vi "Lot_Unload.vi"(8 "error in (no error)":errorcluster, 11 "LotData in":refnum<class "LotData.lvclass">) -> (0 "error out":errorcluster, 3 "LotData out":refnum<class "LotData.lvclass">)   [LabVIEW 2012, in "LotData.lvclass"]
uses:
  LotData.lvclass
  Controls/TestData.ctl
  Controls/Measurement.ctl
  Controls/WaferTable.ctl
  Controls/LotData_Current.ctl
  LotData.lvclass/LotData.ctl
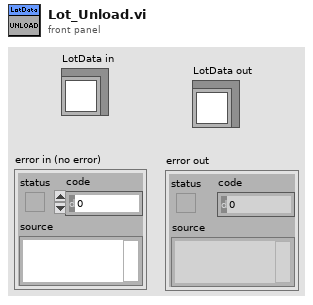
[diagram p1: front panel]
types:
  T1 = cluster{"Area":string, "Wavelength":dbl[], "EL Spectrum":dbl[]}
  T2 = typedef "TestData.ctl" = cluster{"20mA Data":T3, "50mA Data ":T3}
  T3 = typedef "Measurement.ctl" = cluster{"Area":string, "Pad":string, "Current,mA":dbl, "Power":dbl, "WL":dbl, "Voltage":dbl, "Knee Current":dbl, "Reverse":dbl}
  T4 = typedef "LotData.lvclass/LotData_Current.ctl" = cluster{"area":i32, "Data":cluster{"wl":dbl, "power":dbl, "voltage":dbl, "knee":dbl, "reverse":dbl}}
  T5 = typedef "WaferTable.ctl" = string[][]
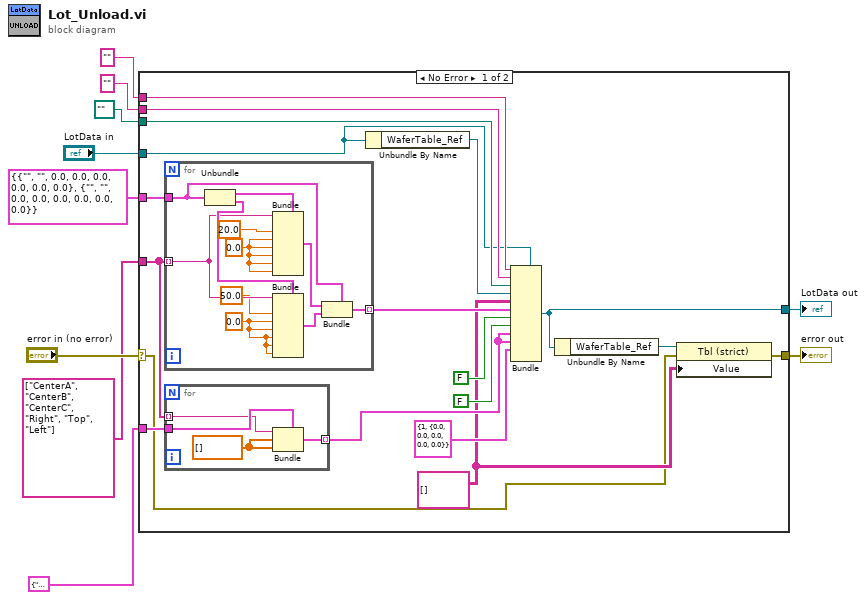
[diagram p0: block diagram]
diagram:
  n1 = case shown="No Error" "error in (no error)" {
    selector: "error in (no error)" -> [w13 w45]
    tunnel: [w11 w45] -> w9
    tunnel: [w12 w44] -> w7
    tunnel: "LotData in" -> [w16 w44]
    tunnel: "" ("Wafer ID") -> [w24 _]
    tunnel: "" ("Type") -> [w23 _]
    tunnel: path "" ("FilePath") -> [w22 _]
    tunnel: T2 {"20mA Data"={"Area"="", "Pad"="", "Current,mA"=0.0, "Power"=0.0, "WL"=0.0, "Voltage"=0.0, "Knee Current"=0.0, "Reverse"=0.0}, "50mA Data "={"Area"="", "Pad"="", "Current,mA"=0.0, "Power"=0.0, "WL"=0.0, "Voltage"=0.0, "Knee Current"=0.0, "Reverse"=0.0}} ("TestData") -> [w21 _]
    tunnel: string[] ["CenterA", "CenterB", "CenterC", "Right", "Top", "Left"] -> [w20 _]
    tunnel: T1 {"Area"="", "Wavelength"=[], "EL Spectrum"=[]} ("Spect") -> [w19 _]
    frame No Error {
      w14 = T5 [] ("WaferTable")
      n2 = for {
        tunnel: w21 -> [w40]
        tunnel: w20 -> [w41] mode=indexing
        tunnel: [w37] -> w28 mode=indexing
        w33 = 0.0 ("Power")
        w35 = 0.0 ("Power")
        n3 = Unbundle(w40) -> ("20mA Data"=w43:T3, "50mA Data"=w42:T3)
        n4 = Bundle(cluster=w43, "Area"=w41, "Current,mA"=20.0, "Power"=w35, "WL"=w35, "Voltage"=w35, "Knee Current"=w35, "Reverse"=w35) -> (w39:T3)  [unwired: 1 in]
        n5 = Bundle(cluster=w42, "Area"=w41, "Current,mA"=50.0, "Power"=w33, "WL"=w33, "Voltage"=w33, "Knee Current"=w33, "Reverse"=w33) -> (w38:T3)  [unwired: 1 in]
        n6 = Bundle(cluster=w40, "20mA Data"=w39, "50mA Data"=w38) -> (w37:T2)
      }
      n7 = for {
        tunnel: w20 -> [w31] mode=indexing
        tunnel: w19 -> [w32]
        tunnel: [w29] -> w25 mode=indexing
        w30 = dbl[] [] ("Wavelength")
        n8 = Bundle(cluster=w32, "Area"=w31, "Wavelength"=w30, "EL Spectrum"=w30) -> (w29:T1)
      }
      n9 = Unbundle By Name(w16) -> ("WaferTable_Ref"=w17:refnum<vi>)
      n10 = Bundle(cluster=w16, w24, w23, w22, w17, w14, w28, FALSE ("Loaded"), FALSE ("Saved"), w25, w25, T4 {"area"=1, "Data"={"wl"=0.0, "power"=0.0, "voltage"=0.0, "knee"=0.0, "reverse"=0.0}} ("Current")) -> (w12:refnum<class "LotData.lvclass">)  [unwired: 1 in]
      n11 = Unbundle By Name(w12) -> ("WaferTable_Ref"=w15:refnum<vi>)
      n12 = property class="Tbl (strict)"(reference=w15, error in=w13, "Value"=w14) -> (error out=w11:errorcluster)  [unwired: 1 out]
    }
    frame Error {
    }
  }
  "error out" <- w9
  "LotData out" <- w7
